vi "BackgateRead.vi"(5 "Backgate Range":dbl, 6 "Backgate Voltage":dbl, 7 "GrphChrt Refnum":refnum<vi>, 8 "error in (no error)":errorcluster, 9 "Path":path, 10 "Ring":u16(ring) items=["Init", "Increment", "End"], 11 "Keithley 2400 Name":refnum<visa-resource-name>="k1") -> (0 "error in (no error) 2":errorcluster, 1 "Resistance":sgl[](array[numeric]), 2 "Cluster":cluster{dbl[], dbl[]}, 3 "Keithley 2400 Name 2":refnum<visa-resource-name>="k1", 4 "Resistance Point":dbl)   [LabVIEW 2019, in "SMU.lvclass"]
uses:
  SMU.lvclass
  <vilib>/Utility/file.llb/Write Delimited Spreadsheet (DBL).vi
  typeDefs/keithleySettings.ctl
panel:
  out "Current":sgl
  out "Voltage":sgl
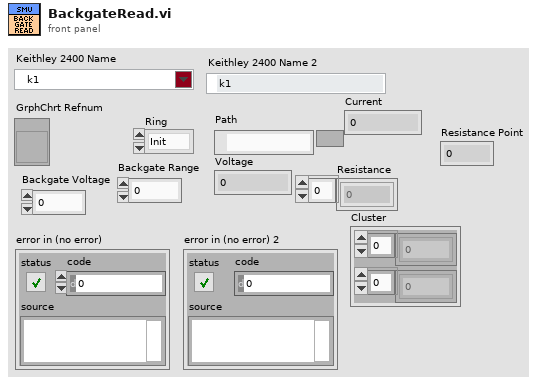
[diagram p1: front panel]
types:
  T1 = typedef "keithleySettings.ctl" = cluster{"Source Compliance (A)":dbl, "Min Voltage (V)":dbl, "Max Voltage (V)":dbl, "Source Mode":u16, "Number of Points":u32}
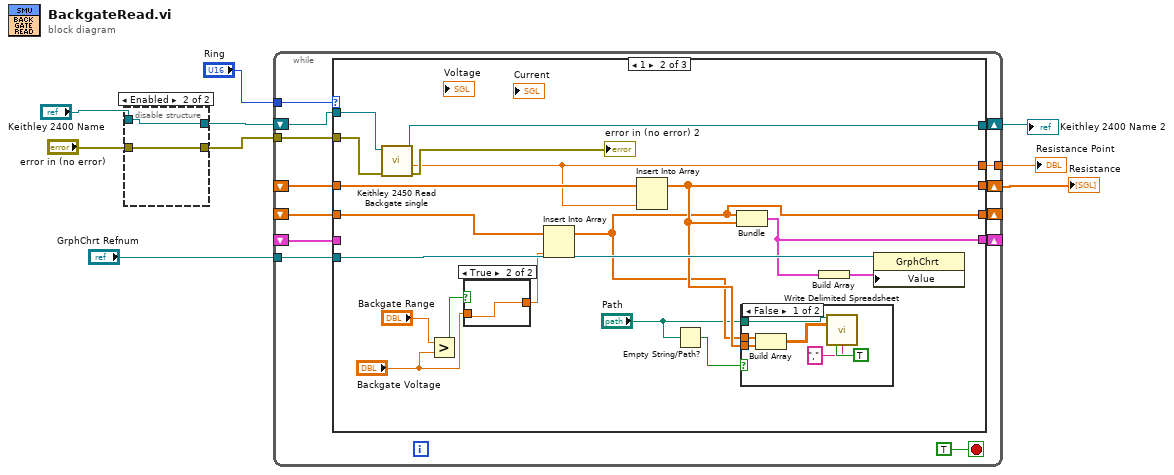
[diagram p0: block diagram]
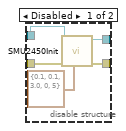
[diagram p2: hidden frame]
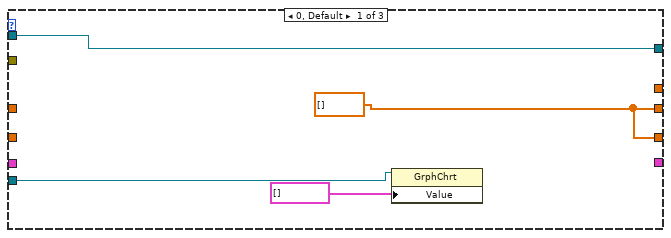
[diagram p3: hidden frame]
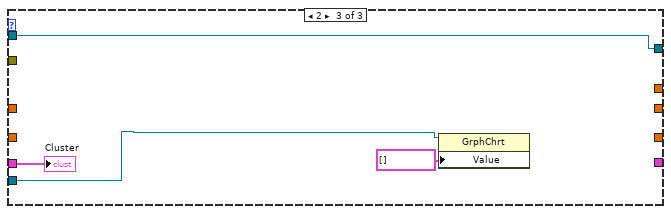
[diagram p6: hidden frame]
diagram:
  n1 = disable-structure shown="Enabled" {
    disable-tunnel: "Keithley 2400 Name" -> [w14 w16]
    disable-tunnel: "error in (no error)" -> [w13 w15]
    disable-tunnel: [w12 w16] -> w5
    disable-tunnel: [w11 w15] -> w4
    frame Disabled {
      n2 = call "SMU2450Init.vi"("Keithley Config"=T1 {"Source Compliance (A)"=0.1, "Min Voltage (V)"=0.1, "Max Voltage (V)"=3.0, "Source Mode"=0, "Number of Points"=5}, "error in (no error)"=w13, "Keithley 2400 Name"=w14) -> ("error out"=w11:errorcluster, "VISA resource name out"=w12:refnum<visa-resource-name>)  [unwired: 7 in]
    }
    frame Enabled {
    }
  }
  n3 = while {
    tunnel: w4 -> [w28]
    tunnel: "GrphChrt Refnum" -> [w27]
    shift-right: [w24] -> _
    shift-left: _ -> [w25]
    shift-right: [w22] -> w2
    shift-left: _ -> [w23]
    tunnel: "Ring" -> [w21]
    shift-right: [w20] -> w3
    shift-left: w5 -> [w29]
    shift-right: [w19] -> _
    shift-left: _ -> [w18]
    tunnel: [w17] -> w1
    stop <- TRUE stop-if-true
    n4 = case shown="1" w21 {
      tunnel: w29 -> [w32 w38 w61]
      tunnel: w28 -> [_ w37 _]
      tunnel: w27 -> [w31 w51 w60]
      tunnel: w25 -> [_ w50 _]
      tunnel: [w33 w46 _] -> w24
      tunnel: w23 -> [_ w49 _]
      tunnel: [w33 w47 _] -> w22
      tunnel: [w32 w35 w61] -> w20
      tunnel: [_ w39 _] -> w19
      tunnel: w18 -> [_ _ w59]
      tunnel: [_ w34 _] -> w17
      frame 0, Default {
        w33 = dbl[] []
        n5 = property class="GrphChrt"(reference=w31, "Value"=cluster{dbl[], dbl[]}[] [] ("appended array")) -> ()  [unwired: 1 in, 2 out]
      }
      frame 1 {
        n6 = call "Keithley 2450 Read Backgate single.vi"("error in (no error)"=w37, "VISA resource name"=w38) -> ("error out (no error) 2"=→"error in (no error) 2":errorcluster, "Resistance (ohm)"=w34:dbl, "VISA resource out"=w35:refnum<visa-resource-name>)  [unwired: 7 in]
        n7 = Greater?(x="Backgate Range", y="Backgate Voltage") -> (0:w40:bool)
        n8 = case shown="True" w40 {
          tunnel: "Backgate Voltage" -> [_ w52]
          tunnel: [_ w52] -> w43
          frame False {
          }
          frame True {
          }
        }
        n9 = Insert Into Array(array=w50, new element=w43) -> (w46:dbl[])  [unwired: 1 in]
        n10 = Insert Into Array(array=w49, new element=w34) -> (w47:dbl[])  [unwired: 1 in]
        n11 = Empty String/Path?(string/path="Path") -> (empty?=w44:bool)
        n12 = Bundle(w46, w47) -> (w39:cluster{dbl[], dbl[]})  [unwired: 1 in]
        n13 = case shown="False" w44 {
          tunnel: w47 -> [w58 _]
          tunnel: w46 -> [w57 _]
          tunnel: "Path" -> [w54 _]
          frame False {
            n14 = Build Array(w57, w58) -> (w56:dbl[][])
            n15 = call-poly <vilib>:"Write Delimited Spreadsheet.vi"("file path (dialog if empty)"=w54, "2D data"=w56, "transpose? (no:F)"=TRUE, "delimiter (\\t)"="," ("delimiter (\\t)")) -> ()  [unwired: 10 in, 2 out]
          }
          frame True {
          }
        }
        n16 = Build Array(w39) -> (w48:cluster{dbl[], dbl[]}[])
        n17 = property class="GrphChrt"(reference=w51, "Value"=w48) -> ()  [unwired: 1 in, 2 out]
      }
      frame 2 {
        n18 = property class="GrphChrt"(reference=w60, "Value"=cluster{dbl[], dbl[]}[] [] ("appended array")) -> ()  [unwired: 1 in, 2 out]
        "Cluster" <- w59
      }
    }
  }
  "Keithley 2400 Name 2" <- w3
  "Resistance" <- w2
  "Resistance Point" <- w1
